vi "VireoTypeRefToVariant.vi"(11 "typeRef":i64) -> (3 "variant":variant)   [LabVIEW 2013]
uses:
  <vilib>/Utility/VariantDataType/TypedefInfo.ctl
  vireo/bin/esh.dll
  <vilib>/Utility/VariantDataType/VariantType.lvlib
  Vireo.framework
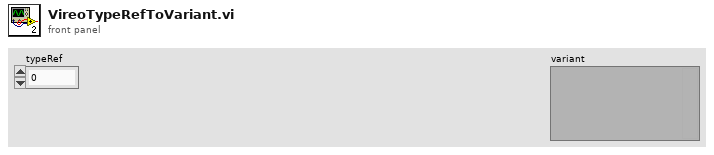
[diagram p1: front panel]
types:
  T1 = typedef "VariantType.lvlib/TypedefInfo.ctl" = cluster{"Name":string, "Timestamp":u32}
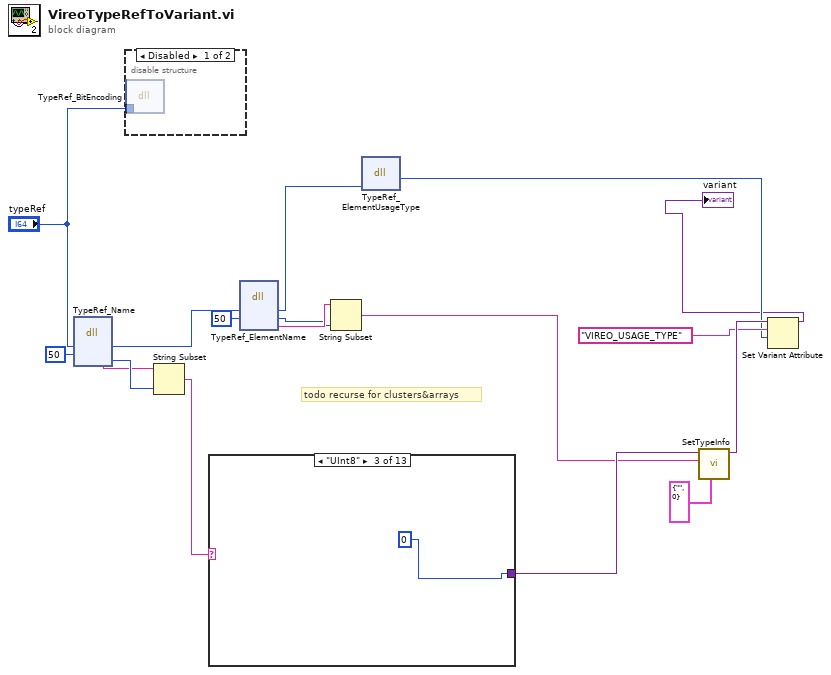
[diagram p0: block diagram]
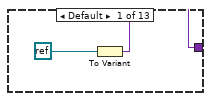
[diagram p2: hidden frame]
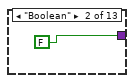
[diagram p3: hidden frame]
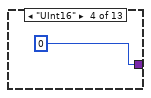
[diagram p4: hidden frame]
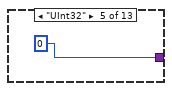
[diagram p5: hidden frame]
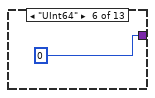
[diagram p6: hidden frame]
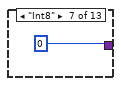
[diagram p7: hidden frame]
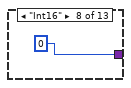
[diagram p8: hidden frame]
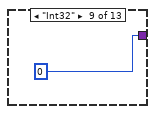
[diagram p9: hidden frame]
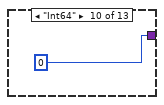
[diagram p10: hidden frame]
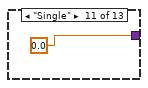
[diagram p11: hidden frame]
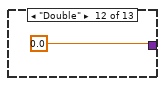
[diagram p12: hidden frame]
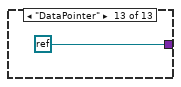
[diagram p13: hidden frame]
diagram:
  # "todo recurse for clusters&arrays"
  n1 = dll-call lib="Macintosh HD/Users/paulaustin/repos/NI_VireoSDK/sample-vis/VireoFunctionNode/Vireo.framework" fn="TypeRef_Name" label="Name"("typeRef"="typeRef", "bufferSize"=50) -> ("typeRef"=w11:i64, "bufferSize"=w17:i32, "name"=w8:string)  [unwired: 5 in, 2 out]
  n2 = disable-structure shown="Disabled" {
    disable-tunnel: "typeRef" -> [w18 _]
    frame Disabled {
      n3 = dll-call lib="E:/dev/vireo/bin/esh.dll" fn="TypeRef_BitEncoding"("typeRef"=w18) -> ()  [unwired: 5 in, 2 out]
    }
    frame Enabled {
    }
  }
  n4 = String Subset(string=w8, length (rest)=w17) -> (substring=w7:string)  [unwired: 1 in]
  n5 = case shown="\"UInt8\"" w7 {
    tunnel: [w19 FALSE u8 0 u16 0 u32 0 u64 0 i8 0 i16 0 0 i64 0 sgl 0.0 0.0 refnum<k0> refnum] -> w10
    frame Default {
      n6 = To Variant(anything=refnum<k0> refnum) -> (Variant=w19:variant)
    }
    frame "Boolean" {
    }
    frame "UInt8" {
    }
    frame "UInt16" {
    }
    frame "UInt32" {
    }
    frame "UInt64" {
    }
    frame "Int8" {
    }
    frame "Int16" {
    }
    frame "Int32" {
    }
    frame "Int64" {
    }
    frame "Single" {
    }
    frame "Double" {
    }
    frame "DataPointer" {
    }
  }
  n7 = dll-call lib="Macintosh HD/Users/paulaustin/repos/NI_VireoSDK/sample-vis/VireoFunctionNode/Vireo.framework" fn="TypeRef_ElementName" label="ElementName"("typeRef"=w11, "bufferSize"=50) -> ("typeRef"=w5:i64, "bufferSize"=w12:i32, "name"=w13:string)  [unwired: 5 in, 2 out]
  n8 = String Subset(string=w13, length (rest)=w12) -> (substring=w9:string)  [unwired: 1 in]
  n9 = dll-call lib="Macintosh HD/Users/paulaustin/repos/NI_VireoSDK/sample-vis/VireoFunctionNode/Vireo.framework" fn="TypeRef_ElementUsageType" label="ElementName"("typeRef"=w5) -> ("return"=w2:i32)  [unwired: 4 in, 2 out]
  n10 = call <vilib>:"SetTypeInfo.vi"("Typedef Info"=T1 {"Name"="", "Timestamp"=0}, "Name"=w9, "Variant"=w10) -> ("Variant Out"=w4:variant)  [unwired: 7 in, 1 out]
  n11 = Set Variant Attribute(Variant=w4, name="VIREO_USAGE_TYPE", value=w2) -> (Variant out=→"variant":variant)  [unwired: 1 in, 2 out]
